vi "Serialize - Text.vi"(8 "error in":errorcluster, 11 "PAS Data in":refnum<class "PAS Data.lvclass">) -> (0 "error out":errorcluster, 2 "Serialized Text":string, 3 "PAS Data out":refnum<class "PAS Data.lvclass">)   [LabVIEW 2016, in "PAS Library.lvlib" / "PAS Data.lvclass"]
uses:
  PAS Data.lvclass
  PAS Data.lvclass/PAS Data.ctl
  Cell/PAS Cell Data.lvclass
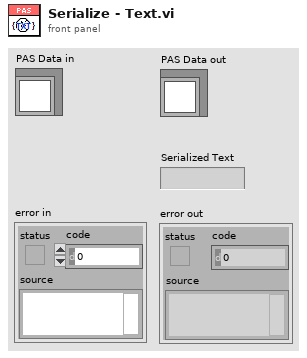
[diagram p1: front panel]
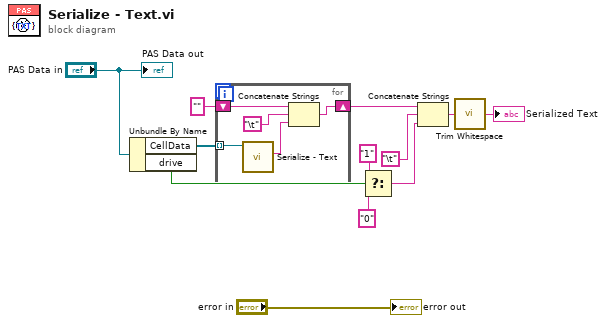
[diagram p0: block diagram]
diagram:
  n1 = Unbundle By Name("PAS Data in") -> ("CellData"=w10:refnum<class "PAS Cell Data.lvclass">[], "drive"=w1:bool)
  n2 = for {
    tunnel: w10 -> [w17] mode=indexing
    shift-right: [w13] -> w6
    shift-left: "" ("Serialized Text") -> [w14]
    n3 = call-dynamic "Serialize - Text.vi"("PAS Cell Data in"=w17) -> ("Serialized Text"=w16:string)  [unwired: 8 in, 2 out]
    n4 = Concatenate Strings(w14, "\t", w16) -> (w13:string)
  }
  n5 = Select(t="1", s=w1, f="0") -> (s? t:f=w4:string)
  n6 = Concatenate Strings(w6, "\t", w4) -> (w3:string)
  n7 = call <vilib>:"Trim Whitespace.vi"("string"=w3) -> ("trimmed string"=→"Serialized Text":string)  [unwired: 1 in]
  "error out" <- "error in"
  "PAS Data out" <- "PAS Data in"
